vi "Alarm Status.vi"(8 "error in (no error)":errorcluster, 10 "Input (0:A)":u16(ring) items=["A", "B", "C", "D"], 11 "VISA resource name":refnum<visa-resource-name>) -> (0 "error out":errorcluster, 1 "Low Alarm Active?":bool, 2 "High Alarm Active?":bool, 3 "VISA resource name out":refnum<visa-resource-name>)   [LabVIEW 2016, in "Lake Shore 336.lvlib"]
doc: "This VI returns the status of the High and Low alarms for the selected input. If an alarm is active, the corresponding indicator will be true."
uses:
  Lake Shore 336.lvlib
  Instance           1 20Saved   Alarm Status .vi
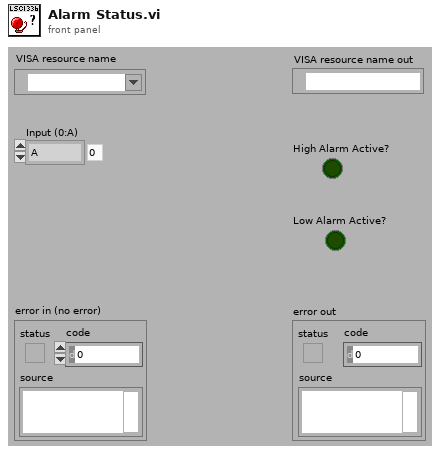
[diagram p1: front panel]
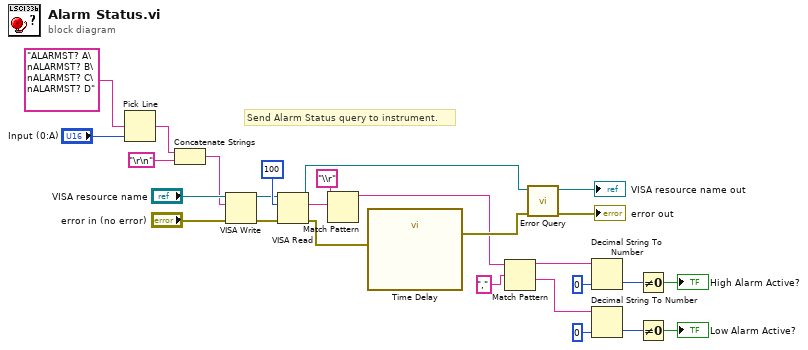
[diagram p0: block diagram]
diagram:
  # "Send Alarm Status query to instrument."
  n1 = Pick Line(multi-line string="ALARMST? A\nALARMST? B\nALARMST? C\nALARMST? D", line index="Input (0:A)") -> (output string=w6:string)  [unwired: 1 in]
  n2 = Concatenate Strings(w6, "\r\n") -> (w4:string)
  n3 = VISA Write(VISA resource name="VISA resource name", write buffer=w4, error in (no error)="error in (no error)") -> (VISA resource name out=w10:refnum<visa-resource-name>, error out=w9:errorcluster)  [unwired: 1 out]
  n4 = VISA Read(VISA resource name=w10, byte count=100, error in (no error)=w9) -> (VISA resource name out=w26:refnum<visa-resource-name>, read buffer=w12:string, error out=w8:errorcluster)  [unwired: 1 out]
  n5 = Match Pattern(string=w12, regular expression="\\r") -> (before substring=w1:string)  [unwired: 1 in, 3 out]
  n6 = call "Time Delay"("error in (no error)"=w8) -> ("error out"=w25:errorcluster)  [unwired: 10 in]
  n7 = Match Pattern(string=w1, regular expression=",") -> (before substring=w16:string, after substring=w2:string)  [unwired: 1 in, 2 out]
  n8 = call "Error Query.vi"("error in (no error)"=w25, "VISA resource name"=w26) -> ("error out"=→"error out":errorcluster, "VISA resource name out"=→"VISA resource name out":refnum<visa-resource-name>)  [unwired: 7 in, 1 out]
  n9 = Decimal String To Number(string=w16, default (0L)=u16 0) -> (number=w19:u16)  [unwired: 1 in, 1 out]
  n10 = Decimal String To Number(string=w2, default (0L)=u16 0) -> (number=w3:u16)  [unwired: 1 in, 1 out]
  n11 = Not Equal To 0?(x=w19) -> (x != 0?=→"High Alarm Active?":bool)
  n12 = Not Equal To 0?(x=w3) -> (x != 0?=→"Low Alarm Active?":bool)
